vi "Main WT1600 v1.vi"(0 "Settings WT1600 ing":T2={"data bits"=8, "parity"=0, "stop bits"=10, "flow control"=0, "baud rate"=8, "COM"=""} {"baud rate" min=5 max=8 step=1; "flow control" items=["None"=0, "XON/XOFF"=1, "RTS/CTS"=2, "DTR/DSR"=4]; "stop bits" items=["1.0"=10, "1.5"=15, "2.0"=20]; "parity" items=["None", "Odd", "Even", "Mark", "Space"]; "data bits" min=5 max=8 step=1}, 1 "STOP":bool, 2 "Range Tors.":bool, 3 "Numeric":i64, 4 "WT1600 configuration":T1={"Wiring A (0: 1P2W)"=0, "Wiring B (0: 1P2W)"=0, "Wiring C (0: 1P2W)"=0, "V Range (12: 1000)"=12, "Element (0: All)"=0, "Element (0: All) 2"=0, "A Range (9: 5A)"=9, "A Sensor Ratio(mV/A) (10.0000) "=10.0, "Zero Cross Filter (0: OFF)"=0, "Line Filter (0: OFF)"=0, "PT Ratio (1.0000)"=1.0, "Scaling (F: OFF)"=FALSE, "CT Ratio (1.0000)"=1.0, "Scaling Factor (1.0000)"=1.0, "Element (0: All) 3"=0, "Display Format (0: Numeric)"=0, "Normal Item Amount (1: 4)"=1, "Harmonics Item Amount (1: 4)"=1, "Average Type (0: OFF)"=0, "Average Count (2: 8)"=2} {"Average Count (2: 8)" items=["2", "4", "8", "16", "32", "64", "128", "256"]; "Average Type (0: OFF)" items=["OFF", "Linear", "Exponent"]; "Harmonics Item Amount (1: 4)" items=["-", "4", "8", "16", "Single List", "Dual List", "Sigma List"]; "Normal Item Amount (1: 4)" items=["ALL", "4", "8", "16", "42", "78"]; "Display Format (0: Numeric)" items=["Numeric", "Wave", "Bar", "Vector", "Trend", "Numeric & Wave", "Numeric & Bar", "Numeric & Trend", "Wave & Bar", "Wave & Trend", "Bar & Trend", "Information"]; "Element (0: All) 3" items=["All", "Element 1", "Element 2", "Element 3", "Element 4", "Element 5", "Element 6"]; "Scaling Factor (1.0000)" min=0.0001 max=99999.9999 step=0.0001 format="%.4f"; "CT Ratio (1.0000)" min=0.0001 max=99999.9999 step=0.0001 format="%.4f"; "PT Ratio (1.0000)" min=0.0001 max=99999.9999 step=0.0001 format="%.4f"; "Line Filter (0: OFF)" items=["OFF", "500Hz", "5.5kHz"]; "Zero Cross Filter (0: OFF)" items=["OFF", "500Hz"]; "A Sensor Ratio(mV/A) (10.0000)" min=0.0001 max=99999.9999 step=0.0001 format="%.4f"; "A Range (9: 5A)" items=["AUTO", "10 mA", "20 mA", "50 mA", "100 mA", "200 mA", "500 mA", "1 A", "2 A", "5 A", "10 A", "20 A", "50 A", "S-AUTO", "50 mV", "100 mV", "250 mV", "500 mV", "1 V", "2.5 V", "5 V", "10 V"]; "Element (0: All) 2" items=["All", "Element 1", "Element 2", "Element 3", "Element 4", "Element 5", "Element 6"]; "Element (0: All)" items=["All", "Element 1", "Element 2", "Element 3", "Element 4", "Element 5", "Element 6"]; "V Range (12: 1000)" items=["AUTO", "1.5", "3", "6", "10", "15", "30", "60", "100", "150", "300", "600", "1000"]; "Wiring C (0: 1P2W)" items=["1P2W", "1P3W", "3P3W", "3P4W", "3V3A", "NONE"]; "Wiring B (0: 1P2W)" items=["1P2W", "1P3W", "3P3W", "3P4W", "3V3A", "NONE"]; "Wiring A (0: 1P2W)" items=["1P2W", "1P3W", "3P3W", "3P4W", "3V3A"]}, 5 "Refresh":bool, 6 "Clust Refnum":refnum<vi>, 7 "Path":string, 8 "status in":bool, 12 "VISA resource name":refnum<visa-resource-name>) -> (9 "error out":errorcluster, 10 "status out":bool, 11 "VISA resource name 2":refnum<visa-resource-name>, 13 "WT1600 configuration out":T1={"Wiring A (0: 1P2W)"=0, "Wiring B (0: 1P2W)"=0, "Wiring C (0: 1P2W)"=0, "V Range (12: 1000)"=12, "Element (0: All)"=0, "Element (0: All) 2"=0, "A Range (9: 5A)"=9, "A Sensor Ratio(mV/A) (10.0000) "=10.0, "Zero Cross Filter (0: OFF)"=0, "Line Filter (0: OFF)"=0, "PT Ratio (1.0000)"=1.0, "Scaling (F: OFF)"=FALSE, "CT Ratio (1.0000)"=1.0, "Scaling Factor (1.0000)"=1.0, "Element (0: All) 3"=0, "Display Format (0: Numeric)"=0, "Normal Item Amount (1: 4)"=1, "Harmonics Item Amount (1: 4)"=1, "Average Type (0: OFF)"=0, "Average Count (2: 8)"=2} {"Average Count (2: 8)" items=["2", "4", "8", "16", "32", "64", "128", "256"]; "Average Type (0: OFF)" items=["OFF", "Linear", "Exponent"]; "Harmonics Item Amount (1: 4)" items=["-", "4", "8", "16", "Single List", "Dual List", "Sigma List"]; "Normal Item Amount (1: 4)" items=["ALL", "4", "8", "16", "42", "78"]; "Display Format (0: Numeric)" items=["Numeric", "Wave", "Bar", "Vector", "Trend", "Numeric & Wave", "Numeric & Bar", "Numeric & Trend", "Wave & Bar", "Wave & Trend", "Bar & Trend", "Information"]; "Element (0: All) 3" items=["All", "Element 1", "Element 2", "Element 3", "Element 4", "Element 5", "Element 6"]; "Scaling Factor (1.0000)" min=0.0001 max=99999.9999 step=0.0001 format="%.4f"; "CT Ratio (1.0000)" min=0.0001 max=99999.9999 step=0.0001 format="%.4f"; "PT Ratio (1.0000)" min=0.0001 max=99999.9999 step=0.0001 format="%.4f"; "Line Filter (0: OFF)" items=["OFF", "500Hz", "5.5kHz"]; "Zero Cross Filter (0: OFF)" items=["OFF", "500Hz"]; "A Sensor Ratio(mV/A) (10.0000)" min=0.0001 max=99999.9999 step=0.0001 format="%.4f"; "A Range (9: 5A)" items=["AUTO", "10 mA", "20 mA", "50 mA", "100 mA", "200 mA", "500 mA", "1 A", "2 A", "5 A", "10 A", "20 A", "50 A", "S-AUTO", "50 mV", "100 mV", "250 mV", "500 mV", "1 V", "2.5 V", "5 V", "10 V"]; "Element (0: All) 2" items=["All", "Element 1", "Element 2", "Element 3", "Element 4", "Element 5", "Element 6"]; "Element (0: All)" items=["All", "Element 1", "Element 2", "Element 3", "Element 4", "Element 5", "Element 6"]; "V Range (12: 1000)" items=["AUTO", "1.5", "3", "6", "10", "15", "30", "60", "100", "150", "300", "600", "1000"]; "Wiring C (0: 1P2W)" items=["1P2W", "1P3W", "3P3W", "3P4W", "3V3A", "NONE"]; "Wiring B (0: 1P2W)" items=["1P2W", "1P3W", "3P3W", "3P4W", "3V3A", "NONE"]; "Wiring A (0: 1P2W)" items=["1P2W", "1P3W", "3P3W", "3P4W", "3V3A"]}, 14 "Settings WT1600 out":T2={"data bits"=8, "parity"=0, "stop bits"=10, "flow control"=0, "baud rate"=8, "COM"=""} {"baud rate" min=5 max=8 step=1; "flow control" items=["None"=0, "XON/XOFF"=1, "RTS/CTS"=2, "DTR/DSR"=4]; "stop bits" items=["1.0"=10, "1.5"=15, "2.0"=20]; "parity" items=["None", "Odd", "Even", "Mark", "Space"]; "data bits" min=5 max=8 step=1}, 15 "WT1600":bool, 16 "Errori WT1600":i64, 17 "Measure Value":sgl[](array[numeric]) format="%^.3e", 18 "Coppia":dbl, 19 "Velocità":dbl)   [LabVIEW 2016]
panel:
  in  "error out 3":errorcluster
  out "error out 2":errorcluster
  in  "Number of Item (15)":u16=15 min=1 max=255 step=1
  in  "Preset (2: Preset 2)":u16(ring)=2 items=["", "Preset1", "Preset2", "Preset3", "Preset4"]
  in  "termination char\n(0xA = '\\n' = LF)":u8=10 format="%.0x"
  in  "MaxErr WT1600":i64
  # "ON\nOFF"
  # "ON\nOFF"
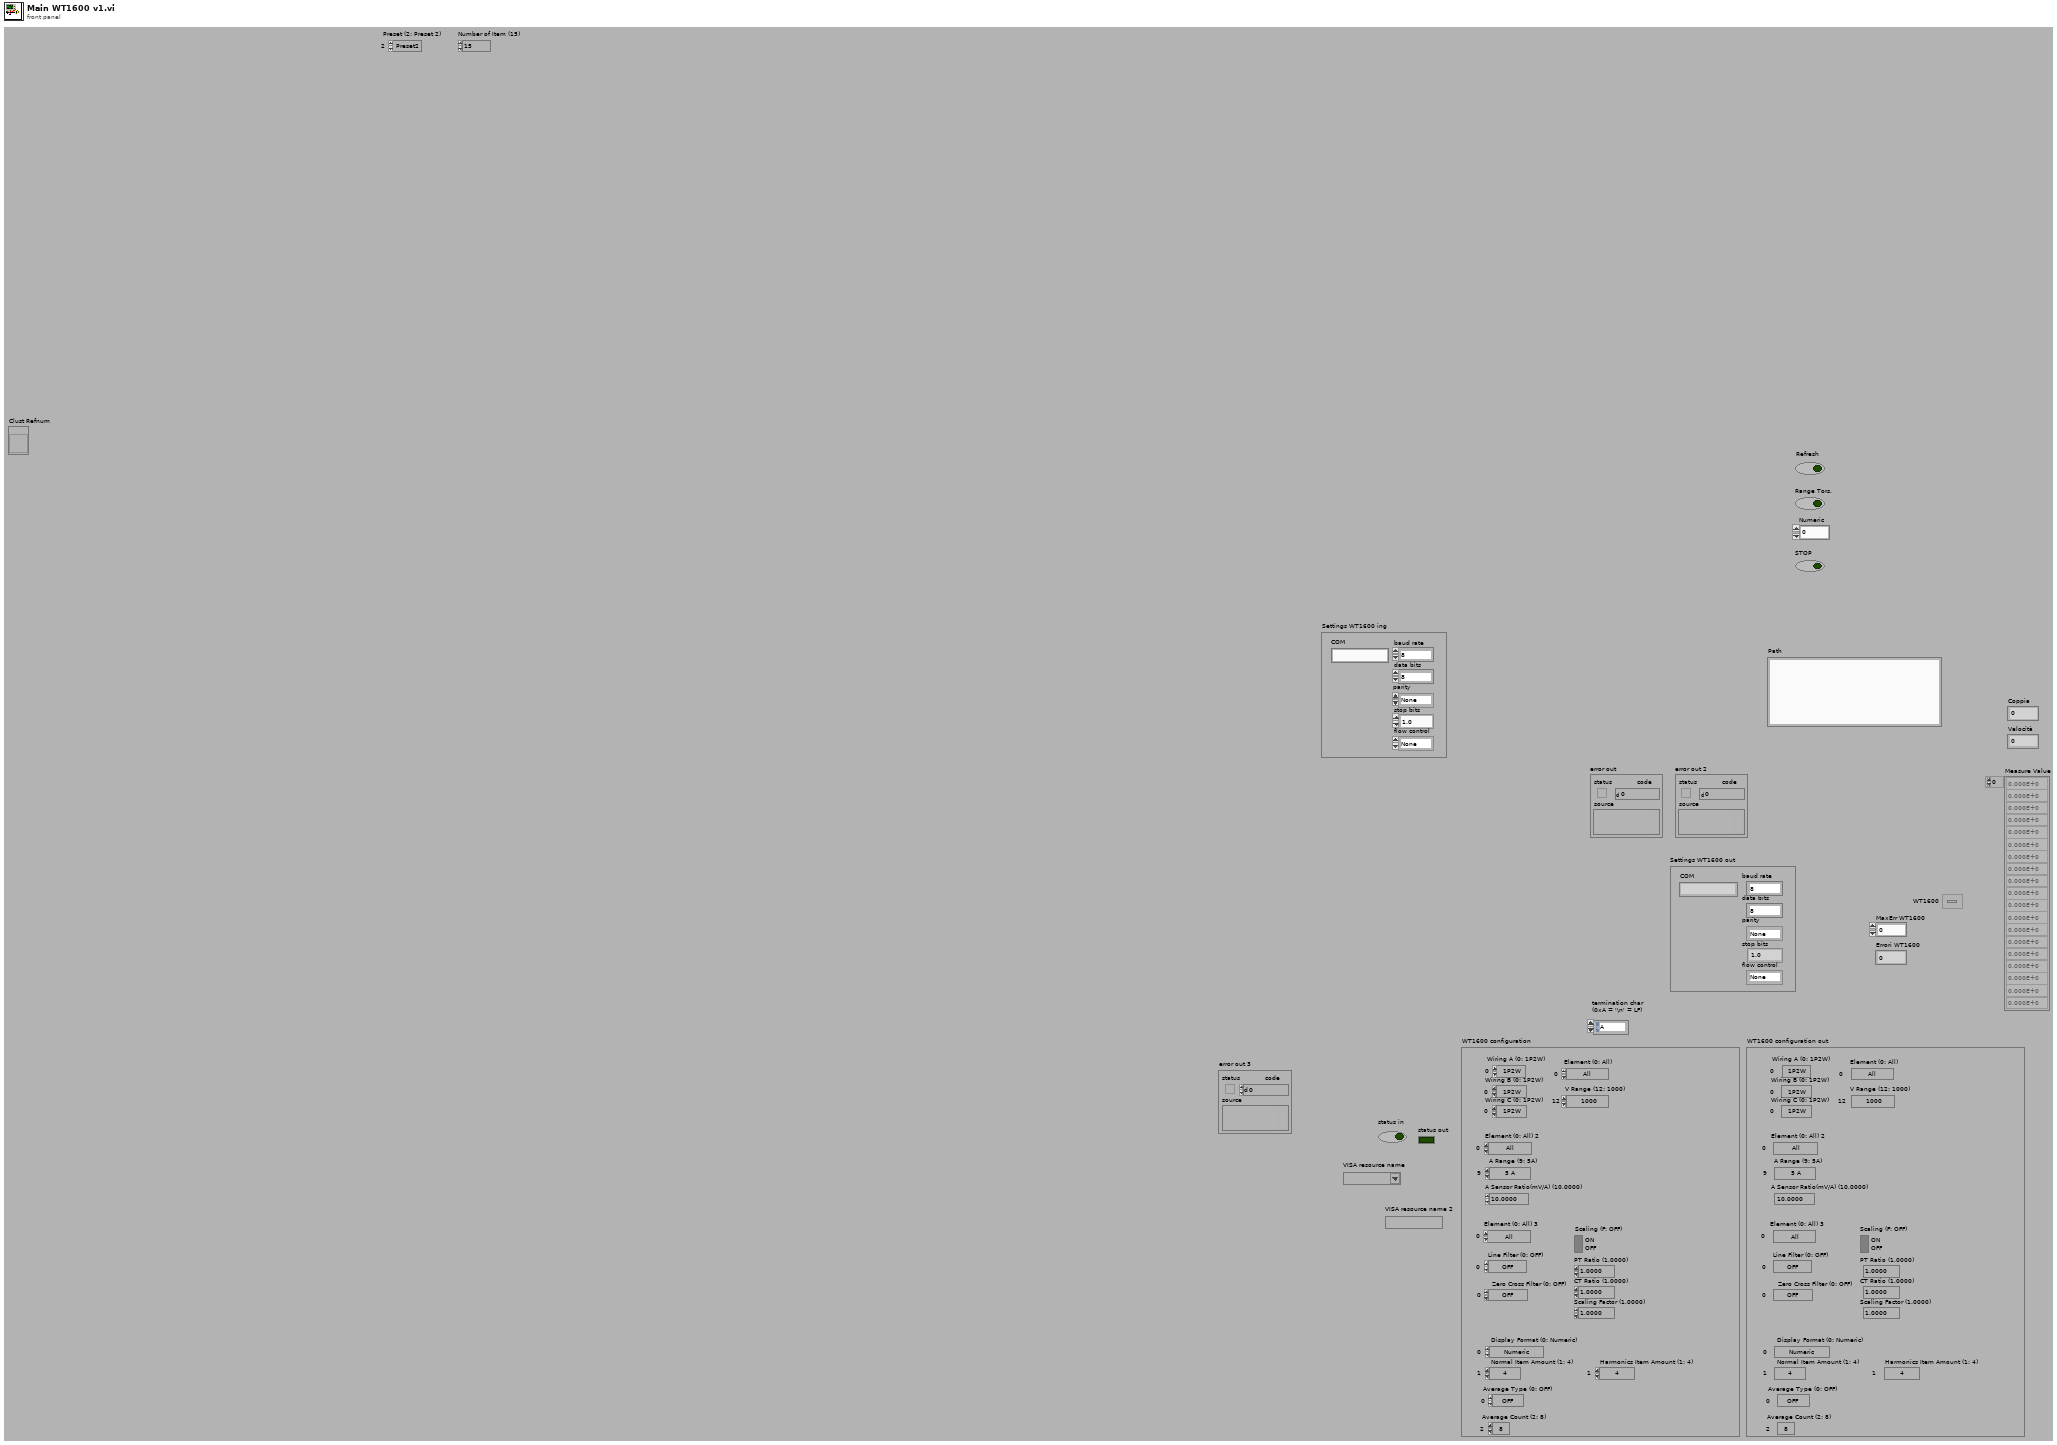
[diagram p1: front panel]
types:
  T1 = cluster{"Wiring A (0: 1P2W)":u16, "Wiring B (0: 1P2W)":u16, "Wiring C (0: 1P2W)":u16, "V Range (12: 1000)":u16, "Element (0: All)":u16, "Element (0: All) 2":u16, "A Range (9: 5A)":u16, "A Sensor Ratio(mV/A) (10.0000) ":dbl, "Zero Cross Filter (0: OFF)":u16, "Line Filter (0: OFF)":u16, "PT Ratio (1.0000)":dbl, "Scaling (F: OFF)":bool, "CT Ratio (1.0000)":dbl, "Scaling Factor (1.0000)":dbl, "Element (0: All) 3":u16, "Display Format (0: Numeric)":u16, "Normal Item Amount (1: 4)":u16, "Harmonics Item Amount (1: 4)":u16, "Average Type (0: OFF)":u16, "Average Count (2: 8)":u16}
  T2 = cluster{"data bits":u16, "parity":u16, "stop bits":u16, "flow control":u16, "baud rate":u16, "COM":string}
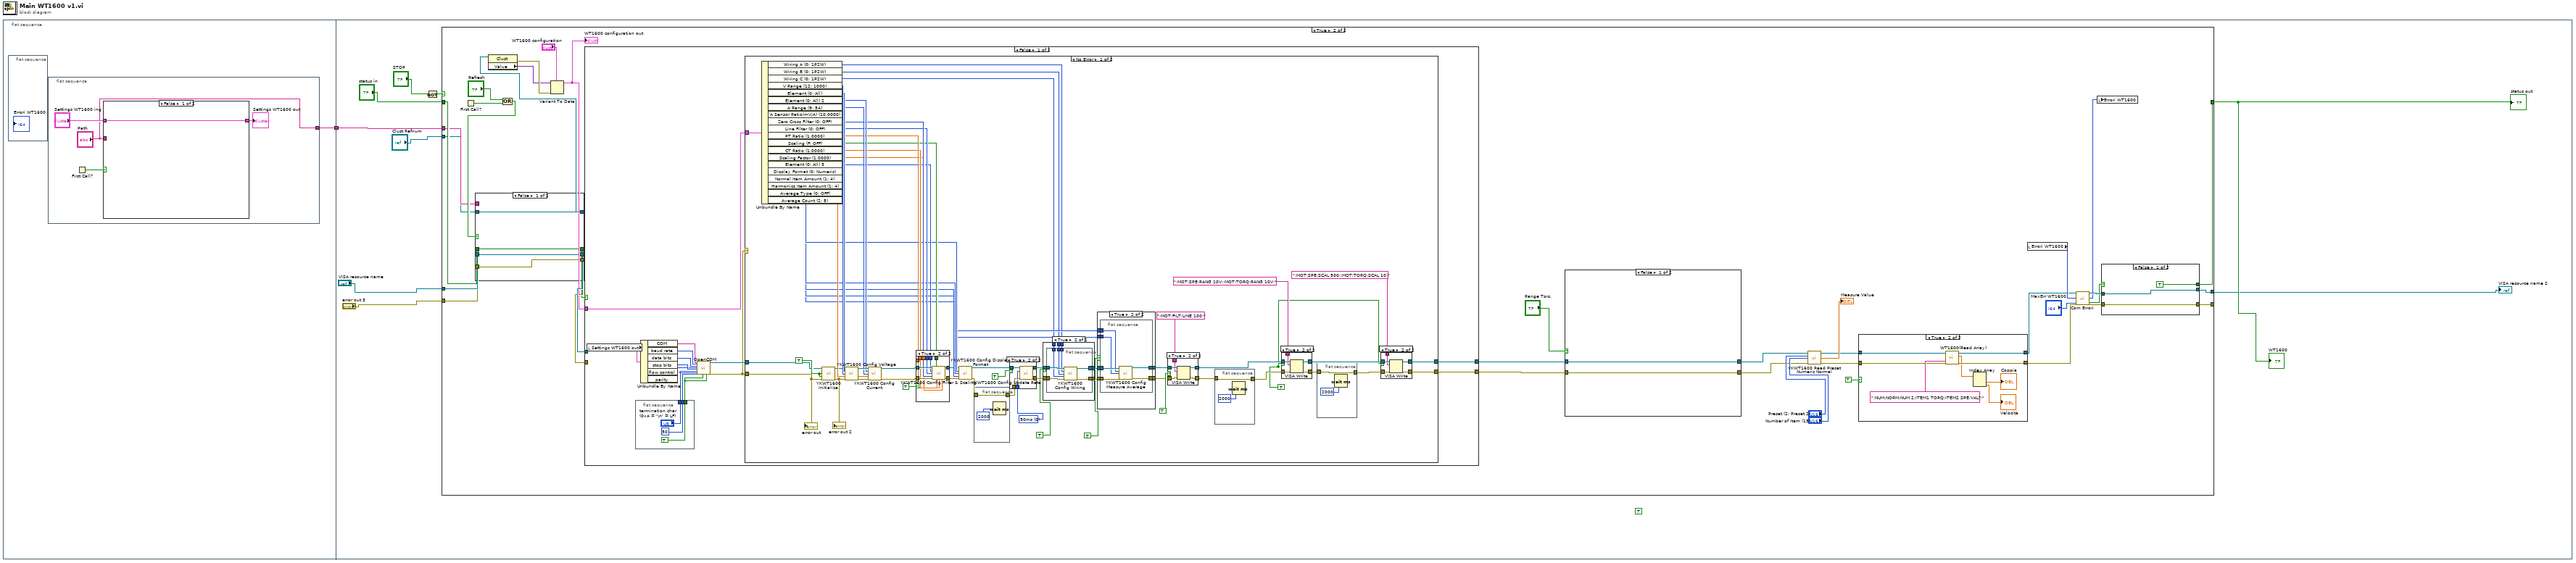
[diagram p0: block diagram]
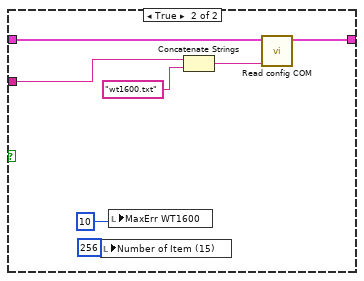
[diagram p2: hidden frame]
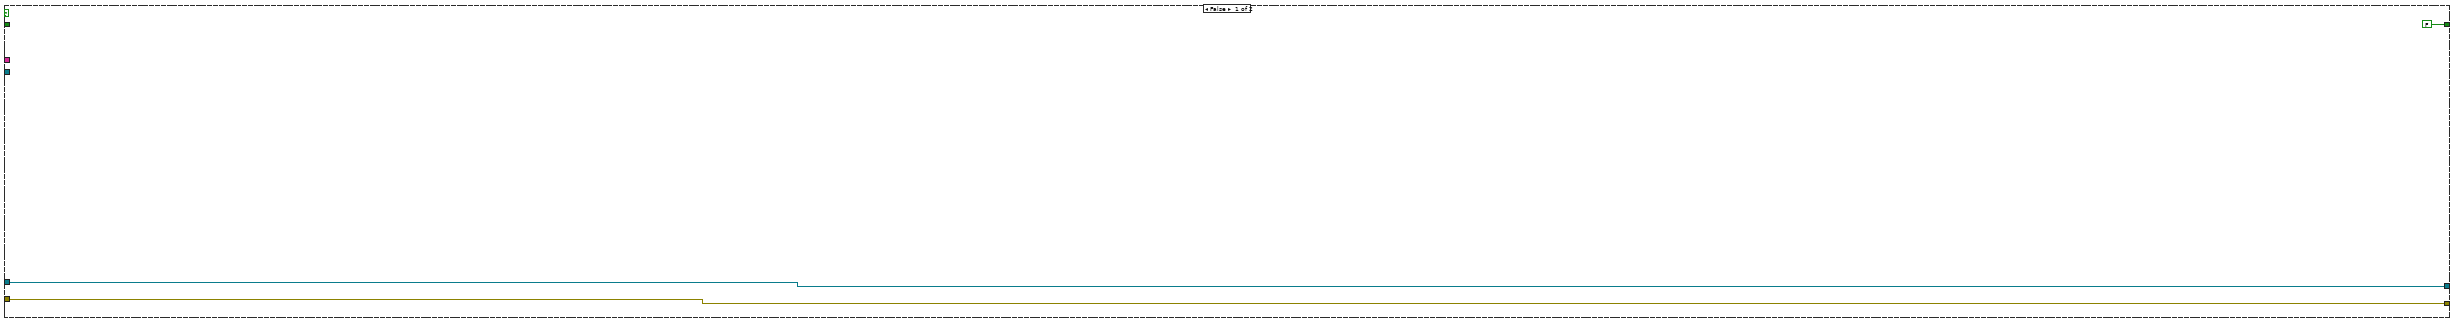
[diagram p3: hidden frame]
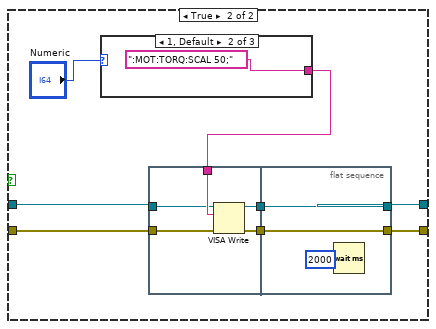
[diagram p4: hidden frame]
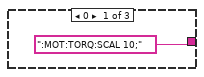
[diagram p5: hidden frame]
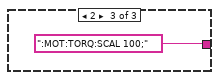
[diagram p6: hidden frame]
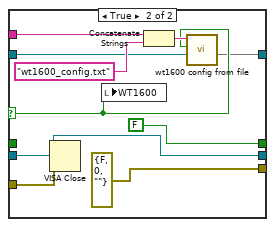
[diagram p8: hidden frame]
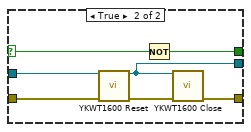
[diagram p18: hidden frame]
diagram:
  n1 = flat-sequence {
    tunnel: [w2] -> w1
    tunnel: w1 -> [w23]
    frame #0 {
      n2 = flat-sequence {
        frame #0 {
        }
      }
      n3 = flat-sequence {
        tunnel: ["Path"] -> w2
        frame #0 {
          n4 = First Call?() -> (First Call?: T/F=w6:bool)
          n5 = case shown="False" w6 {
            tunnel: [w7 w11] -> w4
            tunnel: "Settings WT1600 ing" -> [w7 w12]
            tunnel: "Path" -> [_ w8]
            frame False {
            }
            frame True {
              n6 = local write "Number of Item (15)"(256) -> ()
              n7 = local write "MaxErr WT1600"(10) -> ()
              n8 = Concatenate Strings(w8, "wt1600.txt") -> (w13:string)
              n9 = call "Read config COM.vi"("Path"=w13, "Settings WT1600 ing"=w12) -> ("Settings WT1600 out"=w11:T2)  [unwired: 9 out]
            }
          }
          "Settings WT1600 out" <- w4
        }
      }
    }
    frame #1 {
      (unwired) TRUE
      n10 = Not(x="STOP") -> (.not. x?=w17:bool)
      n11 = case shown="True" w17 {
        tunnel: "status in" -> [_ w54]
        tunnel: "VISA resource name" -> [w25 w56]
        tunnel: [w25 w64] -> w18
        tunnel: [w26 w63] -> _
        tunnel: "error out 3" -> [w26 w55]
        tunnel: [FALSE w62] -> w21
        tunnel: w23 -> [_ w36]
        tunnel: "Clust Refnum" -> [_ w30]
        frame False {
        }
        frame True {
          n12 = First Call?() -> (First Call?: T/F=w41:bool)
          n13 = Compound Arithmetic op=OR("Refresh", w41) -> (w40:bool)
          n14 = case shown="False" w40 {
            selector: w40 -> [_ w103]
            tunnel: [w97 w108] -> w53
            tunnel: w56 -> [w97 w108]
            tunnel: [w98 errorcluster {"status"=FALSE, "code"=0, "source"=""} ("error out")] -> w52
            tunnel: w55 -> [w98 w107]
            tunnel: [w99 FALSE] -> w51
            tunnel: w54 -> [w99 _]
            tunnel: w36 -> [_ w104]
            tunnel: w30 -> [w96 w102]
            tunnel: [w96 w101] -> w29
            frame False {
            }
            frame True {
              n15 = VISA Close(VISA resource name=w108, error in (no error)=w107) -> ()  [unwired: 1 out]
              n16 = local write "WT1600"(w103) -> ()
              n17 = Concatenate Strings(w104, "wt1600_config.txt") -> (w105:string)
              n18 = call "wt1600 config from file.vi"(9:w102, "leggi"=w103, "Path"=w105) -> (1:w101)  [unwired: 1 in, 7 out]
            }
          }
          n19 = property class="Clust"(reference=w29) -> (error out=w35:errorcluster, "Value"=w34:variant)  [unwired: 1 in, 1 out]
          n20 = Variant To Data(error in=w35, type="WT1600 configuration", Variant=w34) -> (data=w27:T1)  [unwired: 1 out]
          "WT1600 configuration out" <- w27
          n21 = case shown="False" w51 {
            tunnel: [w112 w266] -> w31
            tunnel: [w111 w267] -> w32
            tunnel: w52 -> [_ w267]
            tunnel: w53 -> [_ w266]
            tunnel: w27 -> [w115 _]
            frame False {
              n22 = local read "Settings WT1600 out"() -> (w121:T2)
              n23 = flat-sequence {
                tunnel: [TRUE] -> w124
                tunnel: ["termination char\n(0xA = '\\n' = LF)"] -> w123
                tunnel: [50] -> w122
                frame #0 {
                }
              }
              n24 = Unbundle By Name(w121) -> ("COM"=w114:string, "baud rate"=w120:u16, "data bits"=w119:u16, "stop bits"=w118:u16, "flow control"=w116:u16, "parity"=w117:u16)
              n25 = call "OpenCOM.vi"("VISA resource name"=w114, "baud rate (9600)"=w120, "data bits"=w119, "parity"=w117, "stop bits"=w118, "flow control"=w116, "termination char\n(0xA = '\\n' = LF)"=w123, "timeout(ms) solitamente 50ms"=w122, "End Write termination character?"=w124, "End read on termination character?"=w124) -> ("VISA resource name out"=w113:refnum<visa-resource-name>, "error out"=w110:errorcluster)  [unwired: 16 out]
              n26 = case shown="No Error" w110 {
                tunnel: w115 -> [w159 _]
                tunnel: w110 -> [w156 w262]
                tunnel: w113 -> [w154 w261]
                tunnel: [w132 w261] -> w112
                tunnel: [w131 w262] -> w111
                frame No Error {
                  w137 = u16 0 items=["50ms", "100ms", "200ms", "500ms", "1s", "2s", "5s"] ("Update Rate (3: 500ms)")
                  w130 = TRUE
                  w155 = TRUE
                  n27 = Unbundle By Name(w159) -> ("Wiring A (0: 1P2W)"=w153:u16, "Wiring B (0: 1P2W)"=w152:u16, "Wiring C (0: 1P2W)"=w151:u16, "V Range (12: 1000)"=w180:u16, "Element (0: All)"=w179:u16, "Element (0: All) 2"=w178:u16, "A Range (9: 5A)"=w177:u16, "A Sensor Ratio(mV/A) (10.0000)"=w176:dbl, "Zero Cross Filter (0: OFF)"=w175:u16, "Line Filter (0: OFF)"=w174:u16, "PT Ratio (1.0000)"=w173:dbl, "Scaling (F: OFF)"=w170:bool, "CT Ratio (1.0000)"=w172:dbl, "Scaling Factor (1.0000)"=w171:dbl, "Element (0: All) 3"=w169:u16, "Display Format (0: Numeric)"=w168:u16, "Normal Item Amount (1: 4)"=w167:u16, "Harmonics Item Amount (1: 4)"=w166:u16, "Average Type (0: OFF)"=w161:u16, "Average Count (2: 8)"=w160:u16)
                  n28 = call "YKWT1600 Initialize.vi"("VISA session (for class)"=w154, "ID Query (T: Check)"=w155, "Reset (T: Reset)"=w155, "error in (no error)"=w156) -> ("VISA session"=w150:refnum<visa-resource-name>, "error out"=w149:errorcluster)  [unwired: 10 out]
                  "error out 2" <- w149
                  n29 = call "YKWT1600 Config Voltage.vi"("VISA session"=w150, "Element (0: All)"=w179, "V Range (12: 1000)"=w180, "error in (no error)"=w149) -> ("dup VISA session"=w183:refnum<visa-resource-name>, "error out"=w182:errorcluster)  [unwired: 10 out]
                  n30 = call "YKWT1600 Config Current.vi"("VISA session"=w183, "Element (0: All)"=w178, "A Range (9: 5A)"=w177, 9:w176, "error in (no error)"=w182) -> ("dup VISA session"=w181:refnum<visa-resource-name>, "error out"=w125:errorcluster)  [unwired: 9 out]
                  n31 = case shown="True" TRUE {
                    tunnel: w181 -> [w249 w260]
                    tunnel: w125 -> [w248 w259]
                    tunnel: w175 -> [_ w258]
                    tunnel: w174 -> [_ w257]
                    tunnel: w173 -> [_ w256]
                    tunnel: w172 -> [_ w255]
                    tunnel: w171 -> [_ w254]
                    tunnel: w170 -> [_ w253]
                    tunnel: w169 -> [_ w252]
                    tunnel: [w249 w251] -> w165
                    tunnel: [w248 w250] -> w126
                    frame False {
                    }
                    frame True {
                      n32 = call "YKWT1600 Config Filter & Scaling.vi"("VISA session"=w260, "Scaling (F: OFF)"=w253, "Element (0: All)"=w252, "Line Filter (0: OFF)"=w257, "WT 1600 Zero Cross Filter (0: OFF)"=w258, "error in (no error)"=w259, "PT Ratio (1.0000)"=w256, "CT Ratio (1.0000)"=w255, "Scaling Factor (1.0000)"=w254) -> ("dup VISA session"=w251:refnum<visa-resource-name>, "error out"=w250:errorcluster)  [unwired: 2 in, 3 out]
                    }
                  }
                  n33 = call "YKWT1600 Config Display Format.vi"("VISA session"=w165, "Display Format (0: Numeric)"=w168, "Normal Item Amount (1: 4)"=w167, "Harmonics Item Amount (1: 4)"=w166, "error in (no error)"=w126) -> ("dup VISA session"=w141:refnum<visa-resource-name>, "error out"=w142:errorcluster)  [unwired: 9 out]
                  n34 = flat-sequence {
                    tunnel: w142 -> [w231]
                    tunnel: [w231] -> w139
                    frame #0 {
                      n35 = Wait (ms)(milliseconds to wait=2000) -> ()  [unwired: 1 out]
                    }
                  }
                  n36 = case shown="True" TRUE {
                    tunnel: w141 -> [w215 w220]
                    tunnel: [w215 w219] -> w140
                    tunnel: w139 -> [w214 w218]
                    tunnel: [w214 w217] -> w138
                    tunnel: w137 -> [_ w216]
                    frame False {
                    }
                    frame True {
                      n37 = call "YKWT1600 Config Update Rate.vi"("VISA session"=w220, "Update Rate (3: 500ms)"=w216, "error in (no error)"=w218) -> ("dup VISA session"=w219:refnum<visa-resource-name>, "error out"=w217:errorcluster)  [unwired: 11 out]
                    }
                  }
                  n38 = case shown="True" TRUE {
                    tunnel: [w199 w206] -> w163
                    tunnel: [w198 w205] -> w162
                    tunnel: w153 -> [_ w204]
                    tunnel: w152 -> [_ w203]
                    tunnel: w151 -> [_ w202]
                    tunnel: w140 -> [w199 w201]
                    tunnel: w138 -> [w198 w200]
                    frame False {
                    }
                    frame True {
                      n39 = flat-sequence {
                        tunnel: [w212] -> w206
                        tunnel: [w213] -> w205
                        tunnel: w201 -> [w211]
                        tunnel: w200 -> [w210]
                        tunnel: w202 -> [w207]
                        tunnel: w203 -> [w208]
                        tunnel: w204 -> [w209]
                        frame #0 {
                          n40 = call "YKWT1600 Config Wiring.vi"("VISA session"=w211, "Wiring A (0: 1P2W)"=w209, "Wiring B (0: 1P2W)"=w208, "Wiring C (0: 1P2W)"=w207, "error in (no error)"=w210) -> ("dup VISA session"=w212:refnum<visa-resource-name>, "error out"=w213:errorcluster)  [unwired: 9 out]
                        }
                      }
                    }
                  }
                  n41 = case shown="True" TRUE {
                    tunnel: w163 -> [w185 w191]
                    tunnel: w162 -> [w184 w190]
                    tunnel: w161 -> [_ w189]
                    tunnel: w160 -> [_ w188]
                    tunnel: [w185 w187] -> w148
                    tunnel: [w184 w186] -> w147
                    frame False {
                    }
                    frame True {
                      n42 = flat-sequence {
                        tunnel: w191 -> [w197]
                        tunnel: [w196] -> w187
                        tunnel: w190 -> [w195]
                        tunnel: [w194] -> w186
                        tunnel: w189 -> [w193]
                        tunnel: w188 -> [w192]
                        frame #0 {
                          n43 = call "YKWT1600 Config Measure Average.vi"("VISA session"=w197, "Average Type (0: OFF)"=w193, "Average Count (2: 8)"=w192, "error in (no error)"=w195) -> ("dup VISA session"=w196:refnum<visa-resource-name>, "error out"=w194:errorcluster)  [unwired: 10 out]
                        }
                      }
                    }
                  }
                  n44 = case shown="True" TRUE {
                    tunnel: w148 -> [w242 w247]
                    tunnel: w147 -> [w241 w246]
                    tunnel: [w242 w245] -> w158
                    tunnel: [w241 w244] -> w144
                    tunnel: ":MOT:FILT:LINE 100;" -> [_ w243]
                    frame False {
                    }
                    frame True {
                      n45 = VISA Write(VISA resource name=w247, write buffer=w243, error in (no error)=w246) -> (VISA resource name out=w245:refnum<visa-resource-name>, error out=w244:errorcluster)  [unwired: 1 out]
                    }
                  }
                  n46 = flat-sequence {
                    tunnel: w144 -> [w233]
                    tunnel: [w233] -> w143
                    frame #0 {
                      n47 = Wait (ms)(milliseconds to wait=2000) -> ()  [unwired: 1 out]
                    }
                  }
                  n48 = case shown="True" w130 {
                    tunnel: w158 -> [w235 w240]
                    tunnel: w143 -> [w234 w239]
                    tunnel: [w235 w238] -> w134
                    tunnel: [w234 w237] -> w136
                    tunnel: ":MOT:SPE:RANG 10V;:MOT:TORQ:RANG 10V;" -> [_ w236]
                    frame False {
                    }
                    frame True {
                      n49 = VISA Write(VISA resource name=w240, write buffer=w236, error in (no error)=w239) -> (VISA resource name out=w238:refnum<visa-resource-name>, error out=w237:errorcluster)  [unwired: 1 out]
                    }
                  }
                  n50 = flat-sequence {
                    tunnel: w136 -> [w228]
                    tunnel: [w228] -> _
                    tunnel: [w228] -> w133
                    frame #0 {
                      n51 = Wait (ms)(milliseconds to wait=2000) -> ()  [unwired: 1 out]
                    }
                  }
                  n52 = case shown="True" w130 {
                    tunnel: w134 -> [w222 w227]
                    tunnel: w133 -> [w221 w226]
                    tunnel: [w222 w225] -> w132
                    tunnel: [w221 w224] -> w131
                    tunnel: ":MOT:SPE:SCAL 500;:MOT:TORQ:SCAL 10;" -> [_ w223]
                    frame False {
                    }
                    frame True {
                      n53 = VISA Write(VISA resource name=w227, write buffer=w223, error in (no error)=w226) -> (VISA resource name out=w225:refnum<visa-resource-name>, error out=w224:errorcluster)  [unwired: 1 out]
                    }
                  }
                  "error out" <- w156
                }
                frame Error {
                }
              }
            }
            frame True {
            }
          }
          n54 = case shown="False" "Range Tors." {
            tunnel: w31 -> [w66 w74]
            tunnel: w32 -> [w65 w73]
            tunnel: [w65 w72] -> w37
            tunnel: [w66 w71] -> w38
            frame False {
            }
            frame True {
              n55 = case shown="1, Default" "Numeric" {
                tunnel: [":MOT:TORQ:SCAL 10;" ":MOT:TORQ:SCAL 50;" ":MOT:TORQ:SCAL 100;"] -> w68
                frame 0 {
                }
                frame 1, Default {
                }
                frame 2 {
                }
              }
              n56 = flat-sequence {
                tunnel: w68 -> [w82]
                tunnel: w74 -> [w81]
                tunnel: w73 -> [w80]
                tunnel: [w79] -> w70
                tunnel: [w78] -> w69
                tunnel: [w84] -> w71
                tunnel: [w85] -> w72
                tunnel: w70 -> [w85]
                tunnel: w69 -> [w84]
                frame #0 {
                  n57 = VISA Write(VISA resource name=w81, write buffer=w82, error in (no error)=w80) -> (VISA resource name out=w78:refnum<visa-resource-name>, error out=w79:errorcluster)  [unwired: 1 out]
                }
                frame #1 {
                  n58 = Wait (ms)(milliseconds to wait=2000) -> ()  [unwired: 1 out]
                }
              }
            }
          }
          n59 = call "YKWT1600 Read Preset Numeric Normal.vi"("VISA session"=w38, "Preset (2: Preset 2)"="Preset (2: Preset 2)", "Number of Item (15)"="Number of Item (15)", "error in (no error)"=w37) -> ("dup VISA session"=w47:refnum<visa-resource-name>, "Measure"=→"Measure Value":dbl[], "error out"=w46:errorcluster)  [unwired: 2 in, 7 out]
          n60 = case shown="True" TRUE {
            tunnel: w47 -> [w87 w91]
            tunnel: w46 -> [w86 w90]
            tunnel: [w86 w95] -> w45
            tunnel: [w87 w94] -> w44
            frame False {
            }
            frame True {
              n61 = call "WT1600(Read Array).vi"("Read"=":NUM:NORM:NUM 2;ITEM1 TORQ;ITEM2 SPE;VAL?;", "error in (no error)"=w90, "VISA session"=w91) -> ("error out"=w95:errorcluster, "Measure 2"=w93:dbl[], "dup VISA session"=w94:refnum<visa-resource-name>)  [unwired: 6 out]
              n62 = Index Array(array=w93) -> (element #1=→"Coppia":dbl, element #2=→"Velocità":dbl)  [unwired: 2 in]
            }
          }
          n63 = local read "Errori WT1600"() -> (w59:i64)
          n64 = call "Com Errori.vi"("VISA session"=w44, "Errori in"=w59, "Max Errori"="MaxErr WT1600", "error in (no error)"=w45) -> ("dup VISA session"=w61:refnum<visa-resource-name>, "Errori out"=w58:i64, "Chiudi com"=w28:bool, "error out"=w60:errorcluster)  [unwired: 20 out]
          n65 = local write "Errori WT1600"(w58) -> ()
          n66 = case shown="False" w28 {
            selector: w28 -> [_ w277]
            tunnel: w60 -> [w269 w271]
            tunnel: w61 -> [w270 w274]
            tunnel: [w269 w275] -> w63
            tunnel: [w270 w273] -> w64
            tunnel: [TRUE w276] -> w62
            frame False {
            }
            frame True {
              n67 = call "YKWT1600 Reset.vi"("VISA session"=w274, "error in (no error)"=w271) -> ("dup VISA session"=w273:refnum<visa-resource-name>, "error out"=w272:errorcluster)  [unwired: 12 out]
              n68 = Not(x=w277) -> (.not. x?=w276:bool)
              n69 = call "YKWT1600 Close.vi"("VISA session"=w273, "error in (no error)"=w272) -> ("error out"=w275:errorcluster)  [unwired: 13 out]
            }
          }
        }
      }
      "status out" <- w21
      "VISA resource name 2" <- w18
      "WT1600" <- w21
    }
  }
